vi "Num2Str.vi"(7 "value":dbl) -> (8 "output string":string)   [LabVIEW 2024]
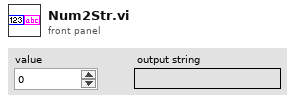
[diagram p1: front panel]
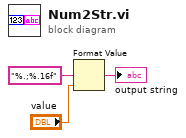
[diagram p0: block diagram]
diagram:
  n1 = Format Value(format string="%.;%.16f", value (0)="value") -> (output string=→"output string":string)  [unwired: 1 in]
